vi "Table to Coordinates.vi"(11 "Waypoint Table":string[][](table)=[["39.485058", "-87.320935", "Facilities Fork"], ["39.483458", "-87.322522", "Cross of Meyers"], ["", "", ""], ["", "", ""], ["\t\t", "", ""]]) -> (3 "Coordinates":T1(array[cluster]))   [LabVIEW 2011]
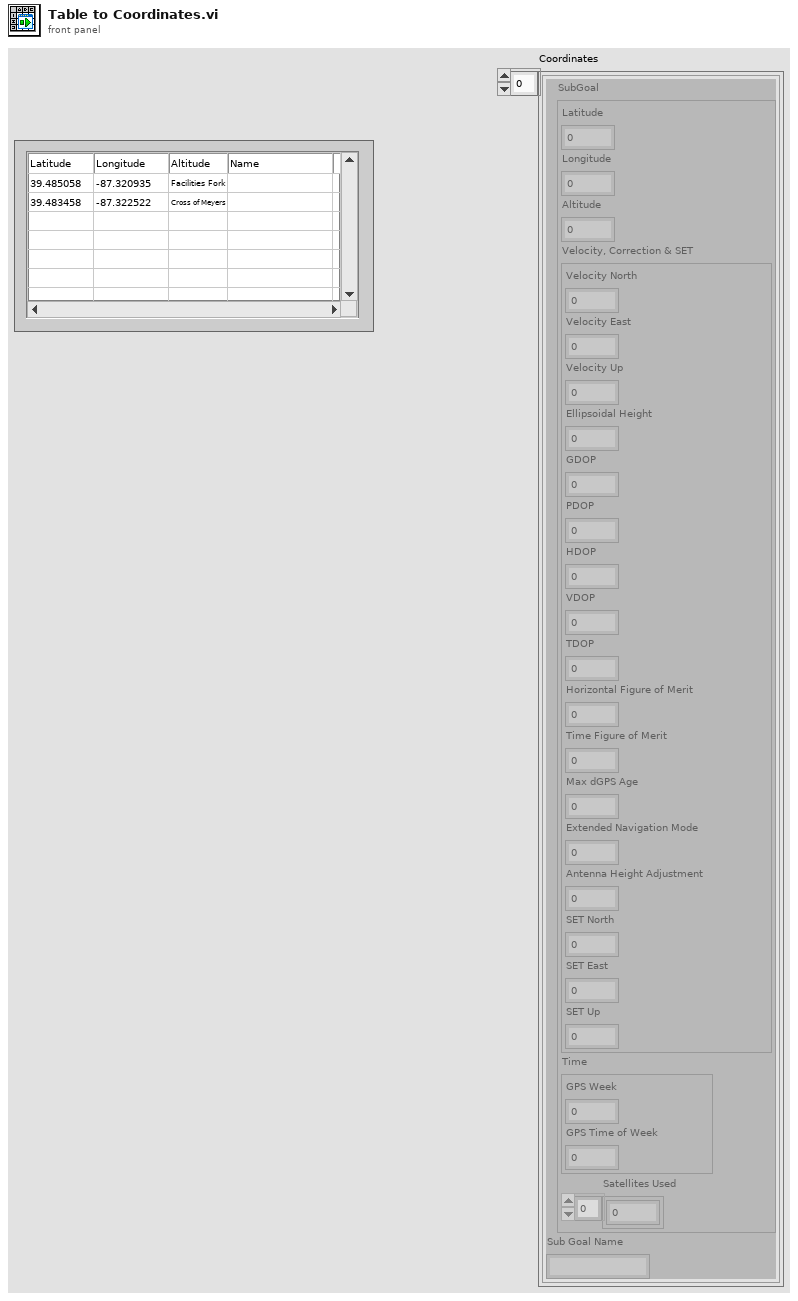
[diagram p1: front panel]
types:
  T1 = cluster{"SubGoal":cluster{"Latitude":dbl, "Longitude":dbl, "Altitude":dbl, "Velocity, Correction & SET":cluster{"Velocity North":dbl, "Velocity East":dbl, "Velocity Up":dbl, "Ellipsoidal Height":dbl, "GDOP":sgl, "PDOP":sgl, "HDOP":sgl, "VDOP":sgl, "TDOP":sgl, "Horizontal Figure of Merit":u8, "Time Figure of Merit":u8, "Max dGPS Age":sgl, "Extended Navigation Mode":u8, "Antenna Height Adjustment ":dbl, "SET North":i32, "SET East":i32, "SET Up":i32}, "Time":cluster{"GPS Week":u16, "GPS Time of Week":sgl}, "Satellites Used":i32[]}, "Sub Goal Name":string}[]
  T2 = cluster{"Latitude":dbl, "Longitude":dbl, "Altitude":dbl, "Velocity, Correction & SET":cluster{"Velocity North":dbl, "Velocity East":dbl, "Velocity Up":dbl, "Ellipsoidal Height":dbl, "GDOP":sgl, "PDOP":sgl, "HDOP":sgl, "VDOP":sgl, "TDOP":sgl, "Horizontal Figure of Merit":u8, "Time Figure of Merit":u8, "Max dGPS Age":sgl, "Extended Navigation Mode":u8, "Antenna Height Adjustment ":dbl, "SET North":i32, "SET East":i32, "SET Up":i32}, "Time":cluster{"GPS Week":u16, "GPS Time of Week":sgl}, "Satellites Used":i32[]}
  T3 = cluster{"SubGoal":cluster{"Latitude":dbl, "Longitude":dbl, "Altitude":dbl, "Velocity, Correction & SET":cluster{"Velocity North":dbl, "Velocity East":dbl, "Velocity Up":dbl, "Ellipsoidal Height":dbl, "GDOP":sgl, "PDOP":sgl, "HDOP":sgl, "VDOP":sgl, "TDOP":sgl, "Horizontal Figure of Merit":u8, "Time Figure of Merit":u8, "Max dGPS Age":sgl, "Extended Navigation Mode":u8, "Antenna Height Adjustment ":dbl, "SET North":i32, "SET East":i32, "SET Up":i32}, "Time":cluster{"GPS Week":u16, "GPS Time of Week":sgl}, "Satellites Used":i32[]}, string}
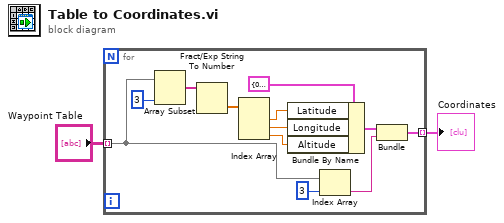
[diagram p0: block diagram]
diagram:
  n1 = for {
    tunnel: "Waypoint Table" -> [w14] mode=indexing
    tunnel: [w3] -> w1 mode=indexing
    n2 = Array Subset(array=w14, length=3) -> (w9:string[])  [unwired: 1 in]
    n3 = Fract/Exp String To Number(string=w9) -> (number=w8:dbl[])  [unwired: 3 in, 1 out]
    n4 = Index Array(array=w8) -> (element #1=w11:dbl, element #2=w10:dbl, element #3=w7:dbl)  [unwired: 3 in]
    n5 = Bundle By Name(cluster=T2 {"Latitude"=0.0, "Longitude"=0.0, "Altitude"=0.0, "Velocity, Correction & SET"={"Velocity North"=0.0, "Velocity East"=0.0, "Velocity Up"=0.0, "Ellipsoidal Height"=0.0, "GDOP"=0.0, "PDOP"=0.0, "HDOP"=0.0, "VDOP"=0.0, "TDOP"=0.0, "Horizontal Figure of Merit"=0, "Time Figure of Merit"=0, "Max dGPS Age"=0.0, "Extended Navigation Mode"=0, "Antenna Height Adjustment "=0.0, "SET North"=0, "SET East"=0, "SET Up"=0}, "Time"={"GPS Week"=0, "GPS Time of Week"=0.0}, "Satellites Used"=[]} ("SubGoal"), "Latitude"=w11, "Longitude"=w10, "Altitude"=w7) -> (w5:T2)
    n6 = Index Array(array=w14, index=3) -> (element=w4:string)
    n7 = Bundle("SubGoal"=w5, w4) -> (w3:T3)  [unwired: 1 in]
  }
  "Coordinates" <- w1
